vi "Write Config.vi"(8 "error in (no error)":errorcluster, 10 "Config":T1={"Process Model"={"Seq Path"=""}, "Break On First Step?"=FALSE, "Break On Step Failure?"=TRUE, "Break On Sequence Failure?"=FALSE, "Tracing Enabled?"=TRUE, "Goto Cleanup on Sequence Failure?"=TRUE}, 11 "teststand-api in":refnum<class "teststand-api.lvclass">) -> (0 "error out":errorcluster, 3 "teststand-api out":refnum<class "teststand-api.lvclass">)   [LabVIEW 2014, in "teststand-api.lvlib" / "teststand-api.lvclass"]
uses:
  teststand-api.lvclass
  Config Argument--cluster.ctl
  Process Model--cluster.ctl
  teststand-api.lvclass/teststand-api.ctl
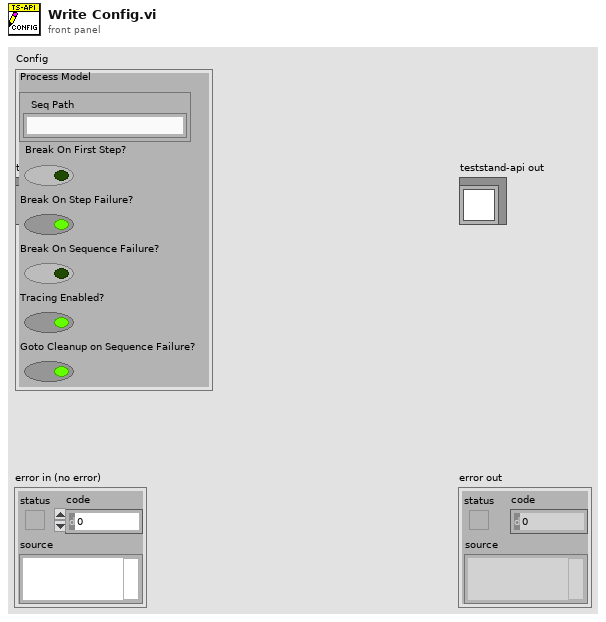
[diagram p1: front panel]
types:
  T1 = typedef "teststand-api.lvlib/teststand-api.lvclass/Config Argument--cluster.ctl" = cluster{"Process Model":T2, "Break On First Step?":bool, "Break On Step Failure?":bool, "Break On Sequence Failure?":bool, "Tracing Enabled?":bool, "Goto Cleanup on Sequence Failure?":bool}
  T2 = typedef "teststand-api.lvlib/teststand-api.lvclass/Process Model--cluster.ctl" = cluster{"Seq Path":string}
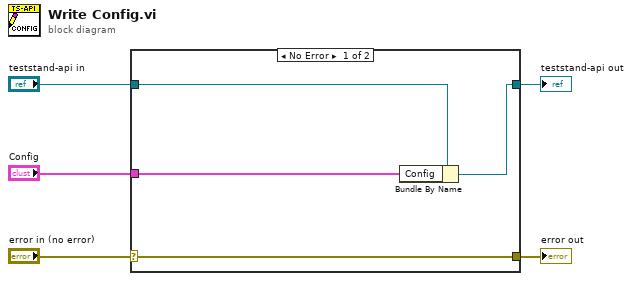
[diagram p0: block diagram]
diagram:
  n1 = case shown="No Error" "error in (no error)" {
    selector: "error in (no error)" -> [w9 w10]
    tunnel: [w9 w10] -> w4
    tunnel: [w7 w11] -> w2
    tunnel: "teststand-api in" -> [w8 w11]
    tunnel: "Config" -> [w6 _]
    frame No Error {
      n2 = Bundle By Name(cluster=w8, "Config"=w6) -> (w7:refnum<class "teststand-api.lvclass">)
    }
    frame Error {
    }
  }
  "error out" <- w4
  "teststand-api out" <- w2
